vi "Connect.vi"(8 "error in (no error)":errorcluster, 10 "Connection String":string, 11 "PostgresqlConnection in":refnum<class "DBC.lvclass">) -> (0 "error out":errorcluster, 3 "PostgresqlConnection out":refnum<class "DBC.lvclass">)   [LabVIEW 2020, in "ORM_DBC_Npgsql.lvlib" / "DBC.lvclass"]
uses:
  DBC.lvclass
  C:/Program Files/National Instruments/LabVIEW 2020/vi.lib/Viviota/shared/ORM_DBC_dotNet.lvlibp/dbcDotNet/ORM_DBC_dotNet.lvclass
  C:/Program Files/National Instruments/LabVIEW 2020/vi.lib/Viviota/shared/ORM.lvlibp/ORM/DbConnection/DbConnection.lvclass
  C:/Program Files/National Instruments/LabVIEW 2020/vi.lib/Viviota/shared/_NET/System.Diagnostics.DiagnosticSource.dll
  Program Files/National Instruments/LabVIEW 2020/vi.lib/Viviota/shared/_NET/System.Diagnostics.DiagnosticSource.dll
  C:/Program Files/National Instruments/LabVIEW 2020/vi.lib/Viviota/shared/_NET/System.Text.Json.dll
  Program Files/National Instruments/LabVIEW 2020/vi.lib/Viviota/shared/_NET/System.Text.Json.dll
  C:/Program Files/National Instruments/LabVIEW 2020/vi.lib/Viviota/shared/_NET/System.Runtime.CompilerServices.Unsafe.dll
  Program Files/National Instruments/LabVIEW 2020/vi.lib/Viviota/shared/_NET/System.Runtime.CompilerServices.Unsafe.dll
  C:/Program Files/National Instruments/LabVIEW 2020/vi.lib/Viviota/shared/_NET/System.Threading.Channels.dll
  Program Files/National Instruments/LabVIEW 2020/vi.lib/Viviota/shared/_NET/System.Threading.Channels.dll
  C:/Program Files/National Instruments/LabVIEW 2020/vi.lib/Viviota/shared/_NET/System.Memory.dll
  Program Files/National Instruments/LabVIEW 2020/vi.lib/Viviota/shared/_NET/System.Memory.dll
  C:/Program Files/National Instruments/LabVIEW 2020/vi.lib/Viviota/shared/_NET/Microsoft.Extensions.Logging.Abstractions.dll
  Program Files/National Instruments/LabVIEW 2020/vi.lib/Viviota/shared/_NET/Microsoft.Extensions.Logging.Abstractions.dll
  C:/Program Files/National Instruments/LabVIEW 2020/vi.lib/Viviota/shared/_NET/System.Threading.Tasks.Extensions.dll
  Program Files/National Instruments/LabVIEW 2020/vi.lib/Viviota/shared/_NET/System.Threading.Tasks.Extensions.dll
  C:/Program Files/National Instruments/LabVIEW 2020/vi.lib/Viviota/shared/_NET/Microsoft.Bcl.AsyncInterfaces.dll
  Program Files/National Instruments/LabVIEW 2020/vi.lib/Viviota/shared/_NET/Microsoft.Bcl.AsyncInterfaces.dll
  C:/Program Files/National Instruments/LabVIEW 2020/vi.lib/Viviota/shared/_NET/Npgsql.dll
  Program Files/National Instruments/LabVIEW 2020/vi.lib/Viviota/shared/_NET/Npgsql.dll
  <vilib>/Viviota/shared/ORM_DBC_dotNet.lvlibp/dbcDotNet/Write connection.vi
  <vilib>/Viviota/shared/ORM.lvlibp/ORM/DbConnection/Write ColumnNameEqualsValueFormat.vi
  <vilib>/Viviota/shared/ORM.lvlibp/ORM/DbConnection/Write ColumnNameFormat.vi
  <vilib>/Viviota/shared/ORM.lvlibp/ORM/DbConnection/Write LastIdentityQuery.vi
  <vilib>/Viviota/shared/ORM.lvlibp/ORM/DbConnection/Write SupportBulkCreate.vi
panel:
  # "Server=localhost;Port=5432;Database=testdb;User Id=postgres;\nPassword=password;"
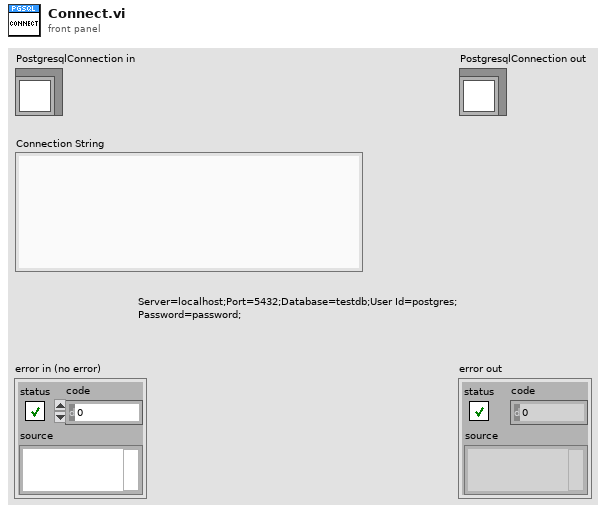
[diagram p1: front panel]
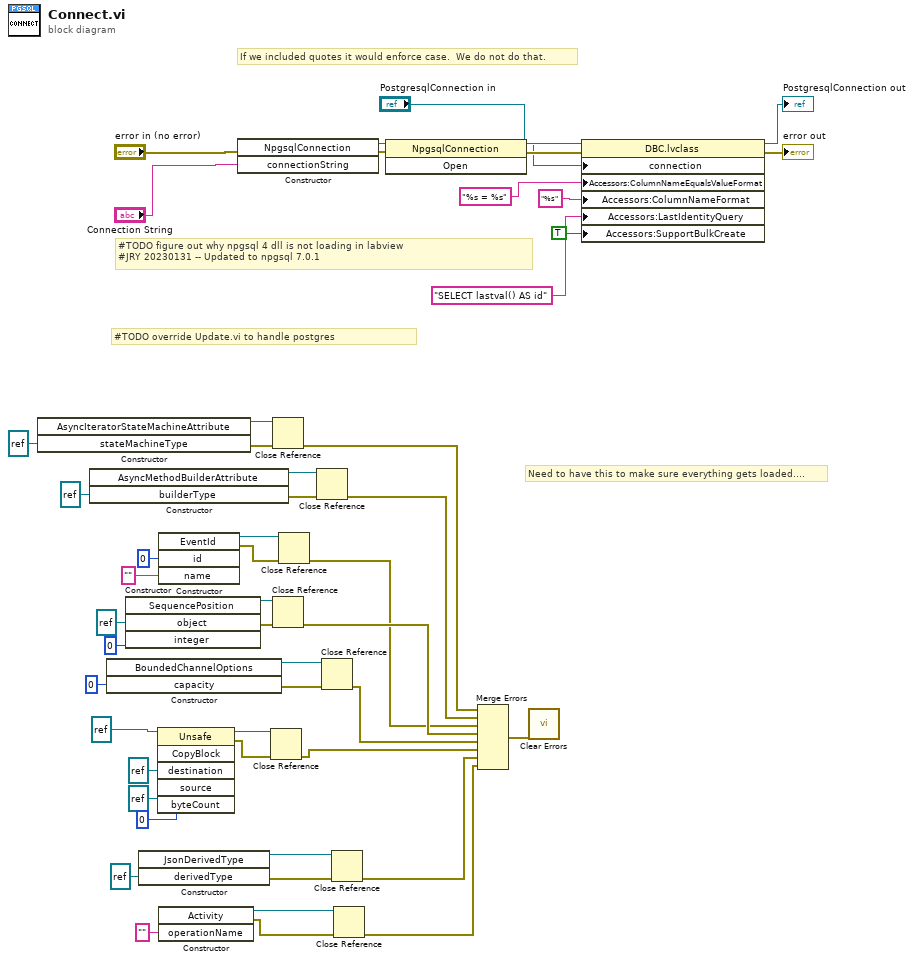
[diagram p0: block diagram]
diagram:
  # "If we included quotes it would enforce case.  We do not do that."
  # "Need to have this to make sure everything gets loaded...."
  # "#TODO override Update.vi to handle postgres"
  # "#TODO figure out why npgsql 4 dll is not loading in labview\n#JRY 20230131 -- Updated to npgsql 7.0.1"
  n1 = constructor class="AsyncIteratorStateMachineAttrib"("stateMachineType"=refnum<k24> refnum) -> (reference out=w40:refnum<k24>, error out=w41:errorcluster)  [unwired: 3 in, 2 out]
  n2 = constructor class="AsyncMethodBuilderAttribute"("builderType"=refnum<k24> refnum) -> (reference out=w37:refnum<k24>, error out=w38:errorcluster)  [unwired: 3 in, 2 out]
  n3 = constructor class="BoundedChannelOptions"("capacity"=0) -> (reference out=w27:refnum<k24>, error out=w26:errorcluster)  [unwired: 3 in, 2 out]
  n4 = constructor class="SequencePosition"("object"=refnum<k24> refnum, "integer"=0) -> (reference out=w30:refnum<k24>, error out=w31:errorcluster)  [unwired: 3 in, 3 out]
  n5 = constructor class="JsonDerivedType"("derivedType"=refnum<k24> refnum) -> (reference out=w16:refnum<k24>, error out=w15:errorcluster)  [unwired: 3 in, 2 out]
  n6 = invoke class="Unsafe" method="CopyBlock"(reference=refnum<k24> refnum ("object"), "destination"=refnum<k24> refnum, "source"=refnum<k24> refnum, "byteCount"=u32 0) -> (reference out=w19:refnum<k24>, error out=w17:errorcluster)  [unwired: 2 in, 4 out]
  n7 = constructor class="EventId"("id"=0, "name"="") -> (reference out=w34:refnum<k24>, error out=w35:errorcluster)  [unwired: 3 in, 3 out]
  n8 = constructor class="Activity"("operationName"="") -> (reference out=w12:refnum<k24>, error out=w13:errorcluster)  [unwired: 3 in, 2 out]
  n9 = constructor class="NpgsqlConnection"(error in="error in (no error)", "connectionString"="Connection String") -> (reference out=w46:refnum<k24>, error out=w42:errorcluster)  [unwired: 2 in, 2 out]
  n10 = Close Reference(reference=w19, error in (no error)=w17) -> (error out=w18:errorcluster)
  n11 = Close Reference(reference=w40, error in (no error)=w41) -> (error out=w4:errorcluster)
  n12 = Close Reference(reference=w30, error in (no error)=w31) -> (error out=w7:errorcluster)
  n13 = Close Reference(reference=w34, error in (no error)=w35) -> (error out=w6:errorcluster)
  n14 = Close Reference(reference=w37, error in (no error)=w38) -> (error out=w5:errorcluster)
  n15 = Close Reference(reference=w27, error in (no error)=w26) -> (error out=w24:errorcluster)
  n16 = Close Reference(reference=w16, error in (no error)=w15) -> (error out=w8:errorcluster)
  n17 = Close Reference(reference=w12, error in (no error)=w13) -> (error out=w9:errorcluster)
  n18 = invoke class="NpgsqlConnection" method="Open"(reference=w46, error in=w42) -> (reference out=w43:refnum<k24>, error out=w45:errorcluster)  [unwired: 1 in, 1 out]
  n19 = Merge Errors(w4, w5, w6, w7, w24, w18, w8, w9) -> (w3:errorcluster)
  n20 = call <vilib>:"Clear Errors.vi"("error in (no error)"=w3) -> ()  [unwired: 5 in, 2 out]
  n21 = property class="DBC.lvclass"(reference="PostgresqlConnection in", error in=w45, "connection"=w43, "Accessors:ColumnNameEqualsValueFormat"="%s = %s" ("ColumnNameFormat"), "Accessors:ColumnNameFormat"="%s" ("ColumnNameFormat"), "Accessors:LastIdentityQuery"="SELECT lastval() AS id" ("LastIdentityQuery"), "Accessors:SupportBulkCreate"=TRUE ("SupportBulkCreate")) -> (reference out=→"PostgresqlConnection out":refnum<class "DBC.lvclass">, error out=→"error out":errorcluster)
